vi "绘制位置虚线.vi"(8 "error in (no error)":errorcluster caption="错误输入（无错误）", 11 "程序 输入":refnum<class "程序.lvclass">) -> (0 "error out":errorcluster caption="错误输出", 2 "new picture":picture, 3 "程序 输出":refnum<class "程序.lvclass">)   [LabVIEW 2020, in "程序.lvclass"]
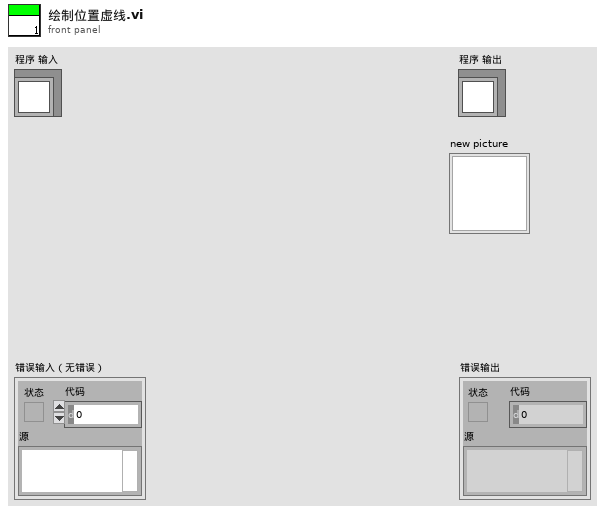
[diagram p1: front panel]
types:
  T1 = cluster{"Width":i16, "Style":enum32{"Solid", "Dash", "Dot", "DashDot", "DashDotDot"}}
  T2 = typedef "LVBoundsTypeDef.ctl" = cluster{"Width":u32, "Height":u32}
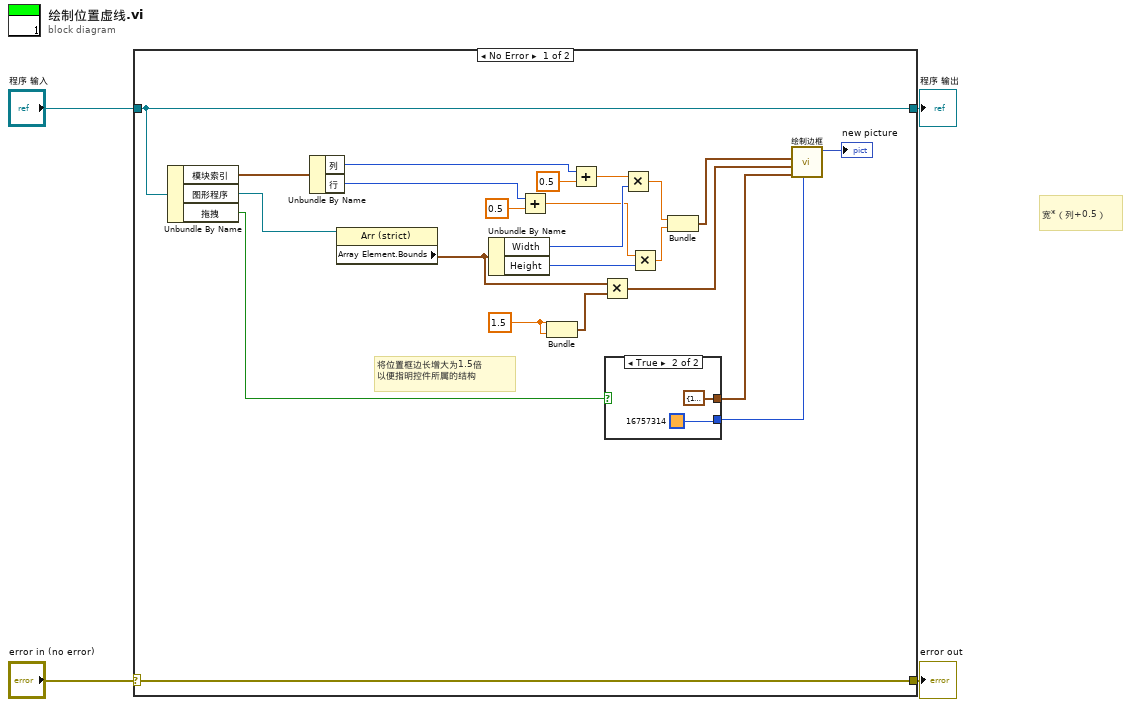
[diagram p0: block diagram]
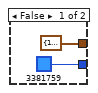
[diagram p2: hidden frame]
diagram:
  # "宽*（列+0.5）"
  n1 = case shown="No Error" "error in (no error)" {
    selector: "error in (no error)" -> [w27 w33]
    tunnel: [w27 w33] -> w3
    tunnel: [w26 w32] -> w1
    tunnel: "程序 输入" -> [w26 w32]
    frame No Error {
      w7 = 1.5 ("y")
      # "将位置框边长增大为1.5倍\n以便指明控件所属的结构"
      n2 = Unbundle By Name(w26) -> ("模块索引"=w25:cluster{"列":u32, "行":u32}, "图形程序"=w24:refnum<vi>, "拖拽"=w18:bool)
      n3 = Unbundle By Name(w25) -> ("列"=w9:u32, "行"=w8:u32)
      n4 = property class="Arr (strict)"(reference=w24) -> ("Array Element.Bounds"=w5:T2)  [unwired: 1 in, 2 out]
      n5 = Unbundle By Name(w5) -> ("Width"=w16:u32, "Height"=w17:u32)
      n6 = Add(x=w8, y=0.5) -> (x+y=w12:dbl)
      n7 = Bundle("y"=w7, "y"=w7) -> (w6:cluster{"y":dbl, "y":dbl})  [unwired: 1 in]
      n8 = Add(x=w9, y=0.5) -> (x+y=w15:dbl)
      n9 = Multiply(x=w5, y=w6) -> (x*y=w20:cluster{dbl, dbl})
      n10 = case shown="True" w18 {
        tunnel: [T1 {"Width"=1, "Style"=enum."Solid"} ("画笔") T1 {"Width"=1, "Style"=enum."Dash"} ("画笔")] -> w23
        tunnel: [u32 3381759 ("颜色") u32 16757314 ("颜色")] -> w22
        frame False {
        }
        frame True {
        }
      }
      n11 = Multiply(x=w15, y=w16) -> (x*y=w11:dbl)
      n12 = Multiply(x=w12, y=w17) -> (x*y=w10:dbl)
      n13 = Bundle(w11, w10) -> (w19:cluster{dbl, dbl})  [unwired: 1 in]
      n14 = call "绘制边框.vi"("颜色"=w22, "画笔"=w23, "大小"=w20, "中心"=w19) -> ("new picture"=→"new picture":picture)  [unwired: 7 in]
    }
    frame Error {
    }
  }
  "error out" <- w3
  "程序 输出" <- w1
